vi "Set Master.vi"(0 "Register Buses":T1[](array[typedef]), 11 "error in":errorcluster) -> (4 "Register Buses (out)":T1[](array[typedef]), 15 "error out":errorcluster)   [LabVIEW 2014, in "ni579x Synchronization v2 Host.lvlib"]
doc: "Set the first FPGA in the array of FPGA VI References as the synchronization master."
uses:
  <instrlib>/ni579x/Synchronization/v2/Host/ni579x Synchronization v2 Host.lvlib
  <instrlib>/_niInstr/Register Bus/v0/Host/Public/Register Bus Session.ctl
  <instrlib>/_niInstr/Register Bus/v0/Host/Private/Session Data.ctl
  <instrlib>/ni579x/Synchronization/v2/Shared/ni579x Synchronization Register Addresses.ctl
  <instrlib>/ni579x/Config/v2/Shared/Types/ni579x Register Bus Subsystem ID.ctl
  <instrlib>/_niInstr/Register Bus/v0/Host/Public/Register Write.ctl
  <instrlib>/ni579x/Config/v2/Shared/ni579x Config v2 Shared.lvlib
  <instrlib>/_niInstr/Register Bus/v0/Host/niInstr Register Bus v0 Host.lvlib
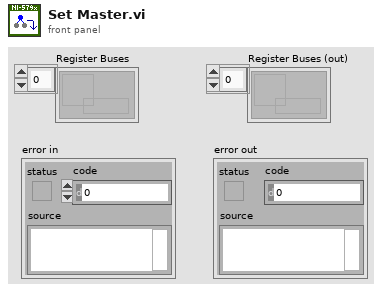
[diagram p1: front panel]
types:
  T1 = typedef "niInstr Register Bus v0 Host.lvlib/Register Bus Session.ctl" = refnum<queue>
  T2 = typedef "niInstr Register Bus v0 Host.lvlib/Register Write.ctl" = cluster{"subsystem":u8, "address":u16, "data":u32}
  T3 = typedef "ni579x Synchronization Register Addresses.ctl" = enum16{"Signature", "Current Version", "Oldest Compatible Version", "Scratch Register", "sync.master", "sync.meas.enable", "sync.meas.ready", "sync.meas.arm", "sync.meas.valid", "sync.meas.value", "sync.cptr.adjust", "sync.cptr.period", "sync.meas.oversample factor"}
  T4 = typedef "ni579x Config v2 Shared.lvlib/ni579x Register Bus Subsystem ID.ctl" = u8
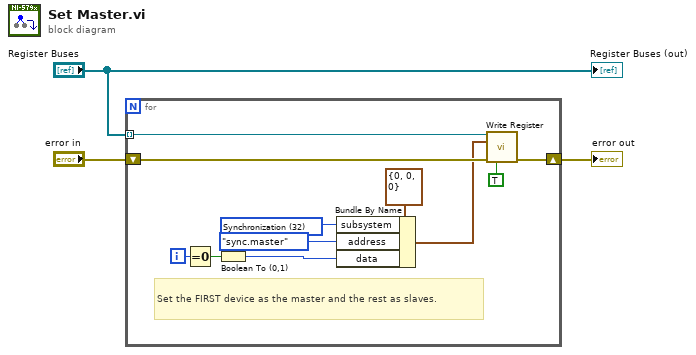
[diagram p0: block diagram]
diagram:
  n1 = for {
    tunnel: "Register Buses" -> [w14] mode=indexing
    shift-right: [w11] -> w1
    shift-left: "error in" -> [w13]
    i -> [w6]
    w8 = T4 32 items=["FAM Register Operation"=0, "User Command"=16, "Synchronization"=32] ("Subsystem ID")
    # "Set the FIRST device as the master and the rest as slaves."
    n2 = Equal To 0?(x=w6) -> (x = 0?=w7:bool)
    n3 = Boolean To (0,1)(Boolean=w7) -> (0, 1=w10:i16)
    n4 = Bundle By Name(cluster=T2 {"subsystem"=0, "address"=0, "data"=0} ("register write"), "subsystem"=w8, "address"=ni579x_Synchronization_Register_Addresses."sync.master" ("Synchronization Registers"), "data"=w10) -> (w5:T2)
    n5 = call <instrlib>:"Write Register.vi"("session in"=w14, "register write"=w5, "error in"=w13, "wait until committed"=TRUE) -> ("error out"=w11:errorcluster)  [unwired: 10 in, 1 out]
  }
  "error out" <- w1
  "Register Buses (out)" <- "Register Buses"
